vi "ArrangeFrontPanel.vi"(8 "error in (no error)":errorcluster, 10 "This VI":refnum<vi>, 11 "MAUI in":refnum<class "MAUI.lvclass">) -> (0 "error out":errorcluster, 3 "MAUI out":refnum<class "MAUI.lvclass">)   [LabVIEW 2016, in "MAUI.lvclass"]
uses:
  MAUI.lvclass
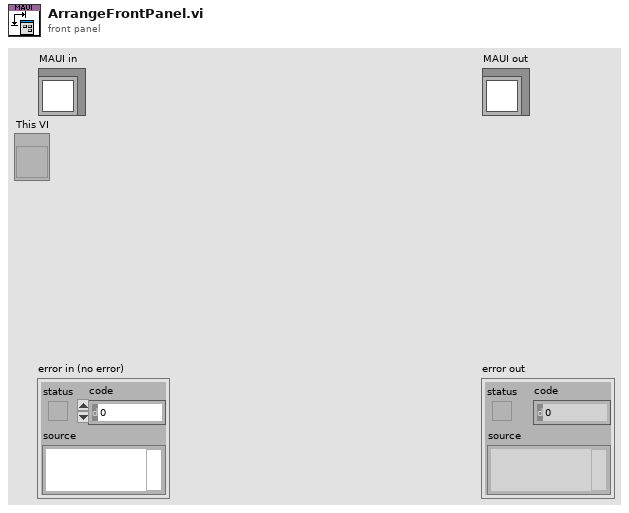
[diagram p1: front panel]
types:
  T1 = typedef "LVRectTypeDef.ctl" = cluster{"Left":i16, "Top":i16, "Right":i16, "Bottom":i16}
  T2 = typedef "LVBoundsTypeDef.ctl" = cluster{"Width":u32, "Height":u32}
  T3 = enum16{"Always On", "Always Off", "Off While Running"}
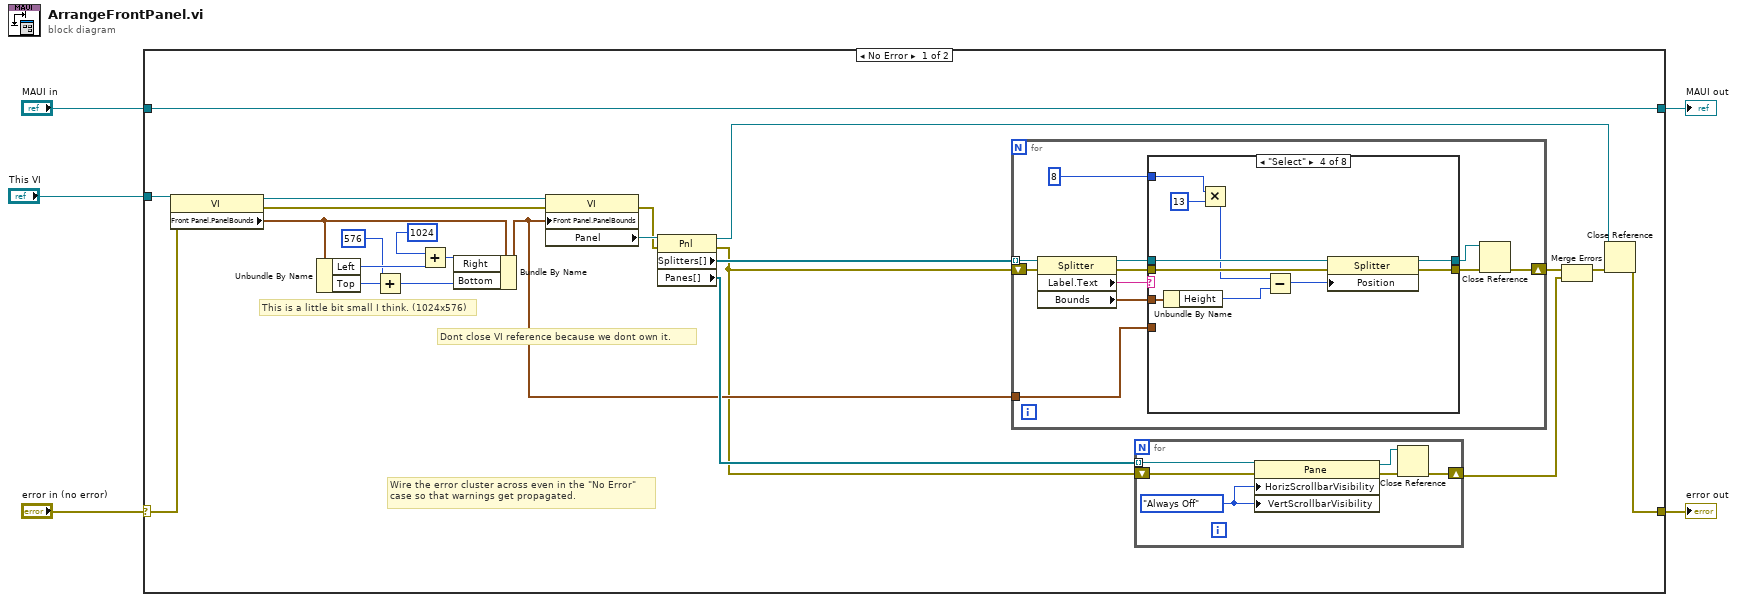
[diagram p0: block diagram]
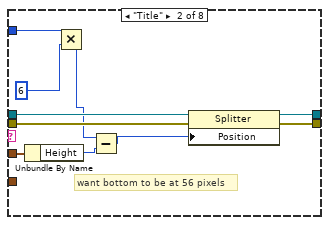
[diagram p3: hidden frame]
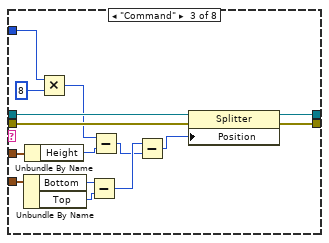
[diagram p4: hidden frame]
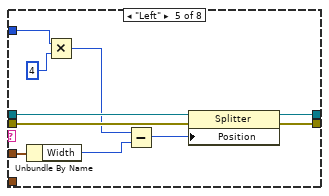
[diagram p5: hidden frame]
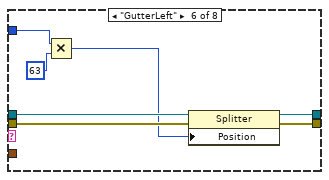
[diagram p6: hidden frame]
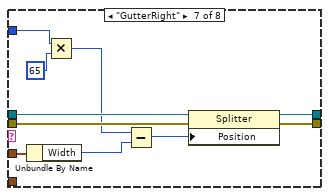
[diagram p7: hidden frame]
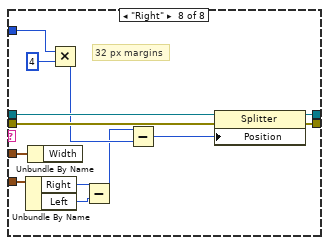
[diagram p8: hidden frame]
diagram:
  n1 = case shown="No Error" "error in (no error)" {
    selector: "error in (no error)" -> [w15 w124]
    tunnel: [w14 w124] -> w4
    tunnel: [w28 w123] -> w2
    tunnel: "MAUI in" -> [w28 w123]
    tunnel: "This VI" -> [w27 _]
    frame No Error {
      # "This is a little bit small I think. (1024x576)"
      # "Dont close VI reference because we dont own it."
      # "Wire the error cluster across even in the \"No Error\"\ncase so that warnings get propagated."
      n2 = property class="VI"(reference=w27, error in=w15) -> (reference out=w21:refnum<vi>, error out=w20:errorcluster, "Front Panel.PanelBounds"=w26:T1)
      n3 = Unbundle By Name(w26) -> ("Left"=w23:i16, "Top"=w24:i16)
      n4 = Add(x=i16 576, y=w24) -> (x+y=w25:i16)
      n5 = Add(x=i16 1024, y=w23) -> (x+y=w22:i16)
      n6 = Bundle By Name(cluster=w26, "Right"=w22, "Bottom"=w25) -> (w10:T1)
      n7 = property class="VI"(reference=w21, error in=w20, "Front Panel.PanelBounds"=w10) -> (error out=w18:errorcluster, "Panel"=w19:refnum<vi>)  [unwired: 1 out]
      n8 = property class="Pnl"(reference=w19, error in=w18) -> (reference out=w16:refnum<vi>, error out=w9:errorcluster, "Splitters[]"=w17:refnum<vi>[], "Panes[]"=w13:refnum<vi>[])
      n9 = for {
        tunnel: w17 -> [w45] mode=indexing
        shift-right: [w39] -> w8
        shift-left: w9 -> [w44]
        tunnel: w10 -> [w35]
        n10 = property class="Splitter"(reference=w45, error in=w44) -> (reference out=w40:refnum<vi>, error out=w42:errorcluster, "Label.Text"=w43:string, "Bounds"=w41:T2)
        n11 = case shown="\"Select\"" w43 {
          tunnel: w42 -> [w47 w56 w71 w81 w91 w98 w108 w119]
          tunnel: w41 -> [_ w54 w69 w79 w89 _ w106 w111]
          tunnel: [w47 w55 w70 w80 w90 w97 w107 w121] -> w38
          tunnel: w40 -> [w46 w57 w72 w82 w92 w99 w109 w120]
          tunnel: [w46 w51 w66 w77 w87 w96 w104 w122] -> w37
          tunnel: 8 -> [_ w50 w65 w75 w85 w95 w102 w118]
          tunnel: w35 -> [_ _ w63 _ _ _ _ w116]
          frame Default {
          }
          frame "Title" {
            # "want bottom to be at 56 pixels"
            n12 = Unbundle By Name(w54) -> ("Height"=w53:u32)
            n13 = Multiply(x=w50, y=6) -> (x*y=w48:i32)
            n14 = Subtract(x=w48, y=w53) -> (x-y=w52:u32)
            n15 = property class="Splitter"(reference=w57, error in=w56, "Position"=w52) -> (reference out=w51:refnum<vi>, error out=w55:errorcluster)
          }
          frame "Command" {
            n16 = Unbundle By Name(w63) -> ("Bottom"=w62:i16, "Top"=w61:i16)
            n17 = Unbundle By Name(w69) -> ("Height"=w68:u32)
            n18 = Multiply(x=w65, y=8) -> (x*y=w67:i32)
            n19 = Subtract(x=w62, y=w61) -> (x-y=w59:i16)
            n20 = Subtract(x=w67, y=w68) -> (x-y=w58:u32)
            n21 = Subtract(x=w59, y=w58) -> (x-y=w60:u32)
            n22 = property class="Splitter"(reference=w72, error in=w71, "Position"=w60) -> (reference out=w66:refnum<vi>, error out=w70:errorcluster)
          }
          frame "Select" {
            n23 = Unbundle By Name(w79) -> ("Height"=w76:u32)
            n24 = Multiply(x=w75, y=13) -> (x*y=w73:i32)
            n25 = Subtract(x=w73, y=w76) -> (x-y=w78:u32)
            n26 = property class="Splitter"(reference=w82, error in=w81, "Position"=w78) -> (reference out=w77:refnum<vi>, error out=w80:errorcluster)
          }
          frame "Left" {
            n27 = Unbundle By Name(w89) -> ("Width"=w86:u32)
            n28 = Multiply(x=w85, y=4) -> (x*y=w83:i32)
            n29 = Subtract(x=w83, y=w86) -> (x-y=w88:u32)
            n30 = property class="Splitter"(reference=w92, error in=w91, "Position"=w88) -> (reference out=w87:refnum<vi>, error out=w90:errorcluster)
          }
          frame "GutterLeft" {
            n31 = Multiply(x=w95, y=63) -> (x*y=w93:i32)
            n32 = property class="Splitter"(reference=w99, error in=w98, "Position"=w93) -> (reference out=w96:refnum<vi>, error out=w97:errorcluster)
          }
          frame "GutterRight" {
            n33 = Unbundle By Name(w106) -> ("Width"=w103:u32)
            n34 = Multiply(x=w102, y=65) -> (x*y=w100:i32)
            n35 = Subtract(x=w100, y=w103) -> (x-y=w105:u32)
            n36 = property class="Splitter"(reference=w109, error in=w108, "Position"=w105) -> (reference out=w104:refnum<vi>, error out=w107:errorcluster)
          }
          frame "Right" {
            # "32 px margins"
            n37 = Unbundle By Name(w116) -> ("Right"=w115:i16, "Left"=w114:i16)
            n38 = Unbundle By Name(w111) -> ()  [unwired: 1 out]
            n39 = Multiply(x=w118, y=4) -> (x*y=w113:i32)
            n40 = Subtract(x=w115, y=w114) -> (x-y=w112:i16)
            n41 = Subtract(x=w112, y=w113) -> (x-y=w110:i32)
            n42 = property class="Splitter"(reference=w120, error in=w119, "Position"=w110) -> (reference out=w122:refnum<vi>, error out=w121:errorcluster)
          }
        }
        n43 = Close Reference(reference=w37, error in (no error)=w38) -> (error out=w39:errorcluster)
      }
      n44 = for {
        tunnel: w13 -> [w34] mode=indexing
        shift-right: [w32] -> w6
        shift-left: w9 -> [w33]
        w29 = T3."Always Off" ("Horizontal Scrollbar Visibility")
        n45 = property class="Pane"(reference=w34, error in=w33, "HorizScrollbarVisibility"=w29, "VertScrollbarVisibility"=w29) -> (reference out=w30:refnum<vi>, error out=w31:errorcluster)
        n46 = Close Reference(reference=w30, error in (no error)=w31) -> (error out=w32:errorcluster)
      }
      n47 = Merge Errors(w8, w6) -> (w7:errorcluster)
      n48 = Close Reference(reference=w16, error in (no error)=w7) -> (error out=w14:errorcluster)
    }
    frame Error {
    }
  }
  "error out" <- w4
  "MAUI out" <- w2
